vi "Dig Freq Meas Check for Multiple Global Channels.vi"(0 "Global Channel In":refnum<k21>, 11 "error in (no error)":errorcluster) -> (4 "Global Channel Out":refnum<k21>, 15 "error out":errorcluster)   [LabVIEW 2021, in "DAQ_Digital Frequency Measurement.lvlib"]
doc: "Checks for the presence of multiple global channels and throws the error if identified"
uses:
  DAQ_Digital Frequency Measurement.lvlib
  <vilib>/Utility/error.llb/Error Cluster From Error Code.vi
  <vilib>/ErrorRing/Error Ring.xnode
  <resource>/objmgr/daqmx.rc
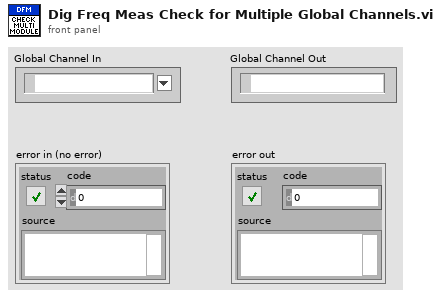
[diagram p1: front panel]
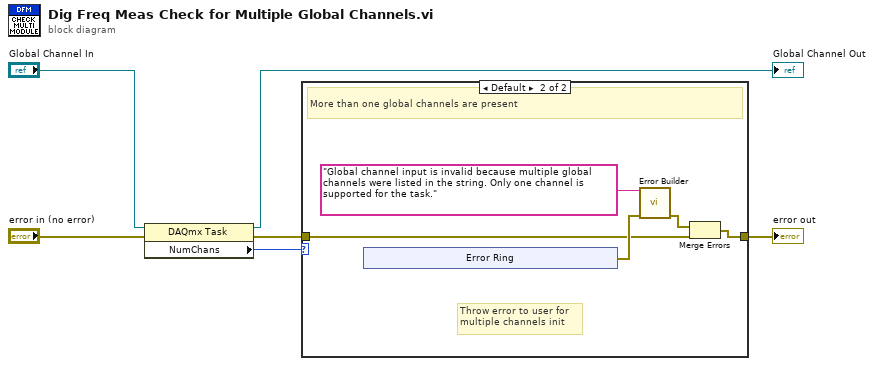
[diagram p0: block diagram]
diagram:
  n1 = property class="DAQmx Task"(reference="Global Channel In", error in="error in (no error)") -> (reference out=→"Global Channel Out":refnum<k21>, error out=w4:errorcluster, "NumChans"=w3:u32)
  n2 = case shown="Default" w3 {
    tunnel: w4 -> [w7 w8]
    tunnel: [w7 w10] -> w1
    frame 1 {
      # "Only 1 channel is present (valid scenario)"
    }
    frame Default {
      # "Throw error to user for \nmultiple channels init"
      # "More than one global channels are present"
      n3 = xnode "Error Ring"() -> ("error out"=w11:errorcluster)
      n4 = call "Error Builder.vi"("Error String"="Global channel input is invalid because multiple global channels were listed in the string. Only one channel is supported for the task." ("error message (\"\")"), "Error In"=w11) -> ("Error Out"=w12:errorcluster)  [unwired: 13 in]
      n5 = Merge Errors(w12, w8) -> (w10:errorcluster)
    }
  }
  "error out" <- w1
